vi "Convert decimal number to hex string.vi"(11 "Decimal number":dbl format="%.4f") -> (3 "Hexadecimal command string":string)   [LabVIEW 2010]
panel:
  out "Decimal number (not rounded)":dbl
  out "Decimal number":i32
  out "Array 2":string[](array[string])
  out "Array":i32[](array[numeric])
  # "set to hex display"
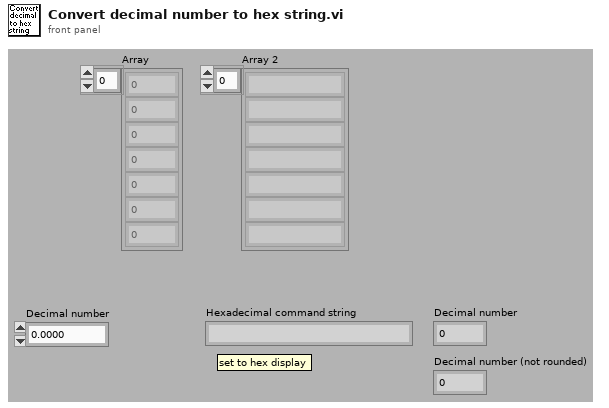
[diagram p1: front panel]
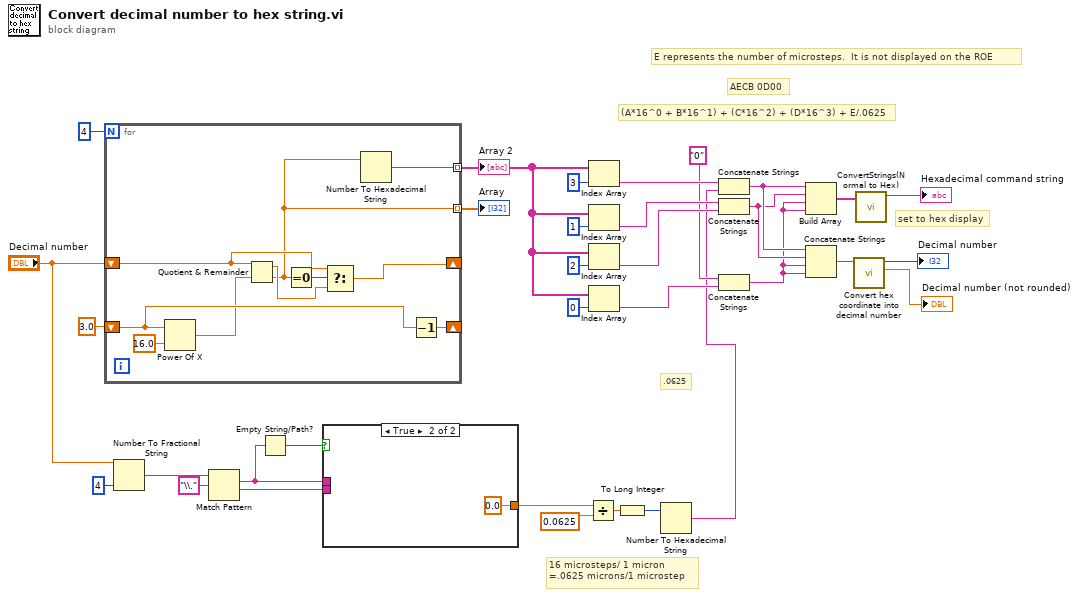
[diagram p0: block diagram]
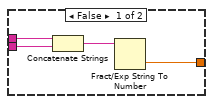
[diagram p2: hidden frame]
diagram:
  # "E represents the number of microsteps.  It is not displayed on the ROE"
  # "16 microsteps/ 1 micron\n=.0625 microns/1 microstep"
  # ".0625"
  # "set to hex display"
  # "(A*16^0 + B*16^1) + (C*16^2) + (D*16^3) + E/.0625"
  # "AECB 0D00"
  n1 = for {
    N: 4 -> [_]
    shift-right: [w41] -> _
    shift-left: 3.0 -> [w42]
    shift-right: [w37] -> _
    shift-left: "Decimal number" -> [w39]
    tunnel: [w36] -> w31 mode=indexing
    tunnel: [w35] -> w26 mode=indexing
    n2 = Power Of X(1:16.0 ("x"), 2:w42) -> (0:w34:dbl)
    n3 = Quotient & Remainder(x=w39, y=w34) -> (x-y*floor(x/y)=w38:dbl, floor(x/y)=w36:dbl)
    n4 = Equal To 0?(x=w36) -> (x = 0?=w40:bool)
    n5 = Select(t=w39, s=w40, f=w38) -> (s? t:f=w37:dbl)
    n6 = Number To Hexadecimal String(2:w36) -> (0:w35:string)  [unwired: 1 out]
    n7 = Decrement(x=w42) -> (x-1=w41:dbl)
  }
  "Array" <- w31
  "Array 2" <- w26
  n8 = Number To Fractional String(number="Decimal number", precision (6)=i16 4) -> (F-format string=w12:string)  [unwired: 2 out]
  n9 = Match Pattern(string=w12, regular expression="\\.") -> (match substring=w9:string, after substring=w8:string)  [unwired: 3 out]
  n10 = Empty String/Path?(string/path=w9) -> (empty?=w10:bool)
  n11 = case shown="True" w10 {
    tunnel: w9 -> [w47 _]
    tunnel: w8 -> [w46 _]
    tunnel: [w44 0.0] -> w7
    frame False {
      n12 = Concatenate Strings(w47, w46) -> (w45:string)
      n13 = Fract/Exp String To Number(string=w45) -> (number=w44:dbl)  [unwired: 4 out]
    }
    frame True {
    }
  }
  n14 = Divide(x=w7, y=0.0625) -> (x/y=w5:dbl)
  n15 = Index Array(array=w26, index=3) -> (element=w24:string)
  n16 = Index Array(array=w26, index=1) -> (element=w23:string)
  n17 = Index Array(array=w26, index=2) -> (element=w22:string)
  n18 = Index Array(array=w26, index=0) -> (element=w21:string)
  n19 = To Long Integer(number=w5) -> (32bit integer=w4:i32)
  n20 = Number To Hexadecimal String(2:w4) -> (0:w2:string)  [unwired: 1 out]
  n21 = Concatenate Strings(w24, w2) -> (w18:string)
  n22 = Concatenate Strings(w23, w22) -> (w17:string)
  n23 = Concatenate Strings("0", w21) -> (w16:string)
  n24 = Build Array(w18, w17, w16, w16) -> (w19:string[])
  n25 = Concatenate Strings(w18, w17, w16, w16) -> (w15:string)
  n26 = call "Convert hex coordinate into decimal number.vi"("Coordinate"=w15) -> ("Decimal number (not rounded)"=→"Decimal number (not rounded)":dbl, "Decimal number (rounded)"=→"Decimal number":i32)  [unwired: 9 out]
  n27 = call "ConvertStrings(Normal to Hex).vi"("Byte array"=w19) -> ("Hexadecimal command string"=→"Hexadecimal command string":string)  [unwired: 10 out]
